vi "First Image Added.vi"(0 "object in":refnum<class "MSC Video Writer.lvclass">, 5 "error in (no error)":errorcluster) -> (14 "object out":refnum<class "MSC Video Writer.lvclass">, 15 "First Image Added":bool, 19 "error out":errorcluster)   [LabVIEW 2014]
uses:
  MSC Video Writer.lvclass
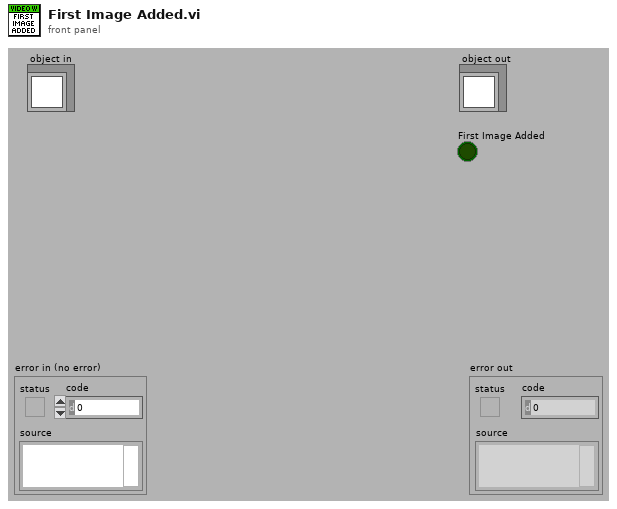
[diagram p1: front panel]
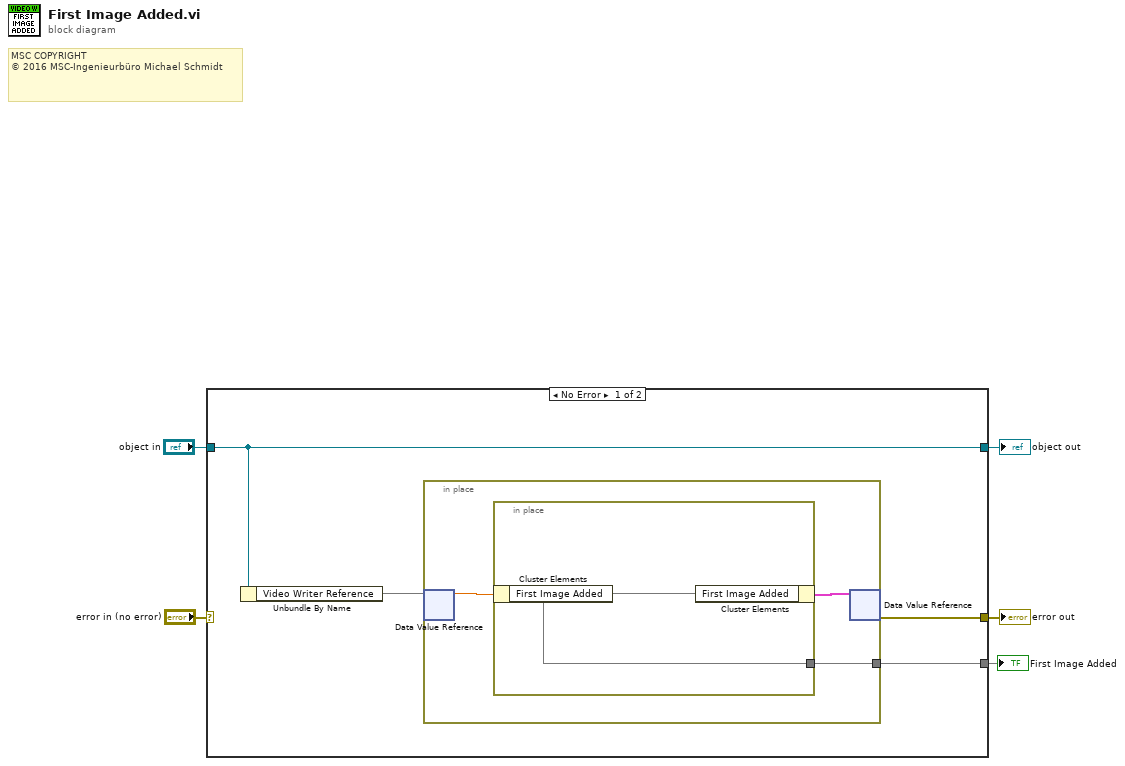
[diagram p0: block diagram]
diagram:
  # "MSC COPYRIGHT\n© 2016 MSC-Ingenieurbüro Michael Schmidt"
  # "MSC COPYRIGHT\n© 2016 MSC-Ingenieurbüro Michael Schmidt"
  n1 = case shown="No Error" "error in (no error)" {
    selector: "error in (no error)" -> [_ w15]
    tunnel: [w8 w15] -> w4
    tunnel: [w9 w14] -> w2
    tunnel: "object in" -> [w9 w14]
    tunnel: [w6 _] -> w1
    frame No Error {
      n2 = Unbundle By Name(w9) -> ("Video Writer Reference"=w7)
      n3 = in-place {
        in-place-border: [w10] -> w6
        n4 = in-place-dvr #1(w7) -> (w11:dbl)  [unwired: 1 out]
        n5 = in-place {
          in-place-border: [w13] -> w10
          n6 = in-place-cluster #2(w11) -> ("First Image Added"=w13)
          n7 = in-place-cluster #2("First Image Added"=w13) -> (w12:cluster{})
        }
        n8 = in-place-dvr #1(w12) -> (w8:errorcluster)  [unwired: 1 out]
      }
    }
    frame Error {
    }
  }
  "error out" <- w4
  "object out" <- w2
  "First Image Added" <- w1
